vi "sumador encoder.vi"() -> ()   [LabVIEW 2025]
panel:
  out "Posición (flancos)":i32
  out "x+y":i32
  out "B":i32
  out "A":i32
  in  "stop":bool
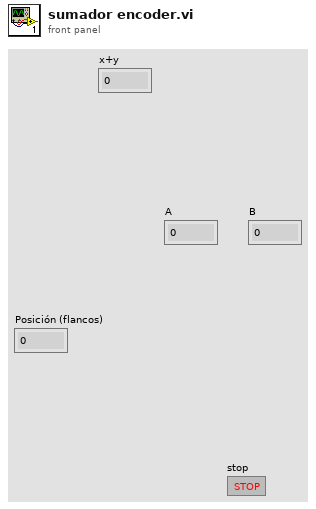
[diagram p1: front panel]
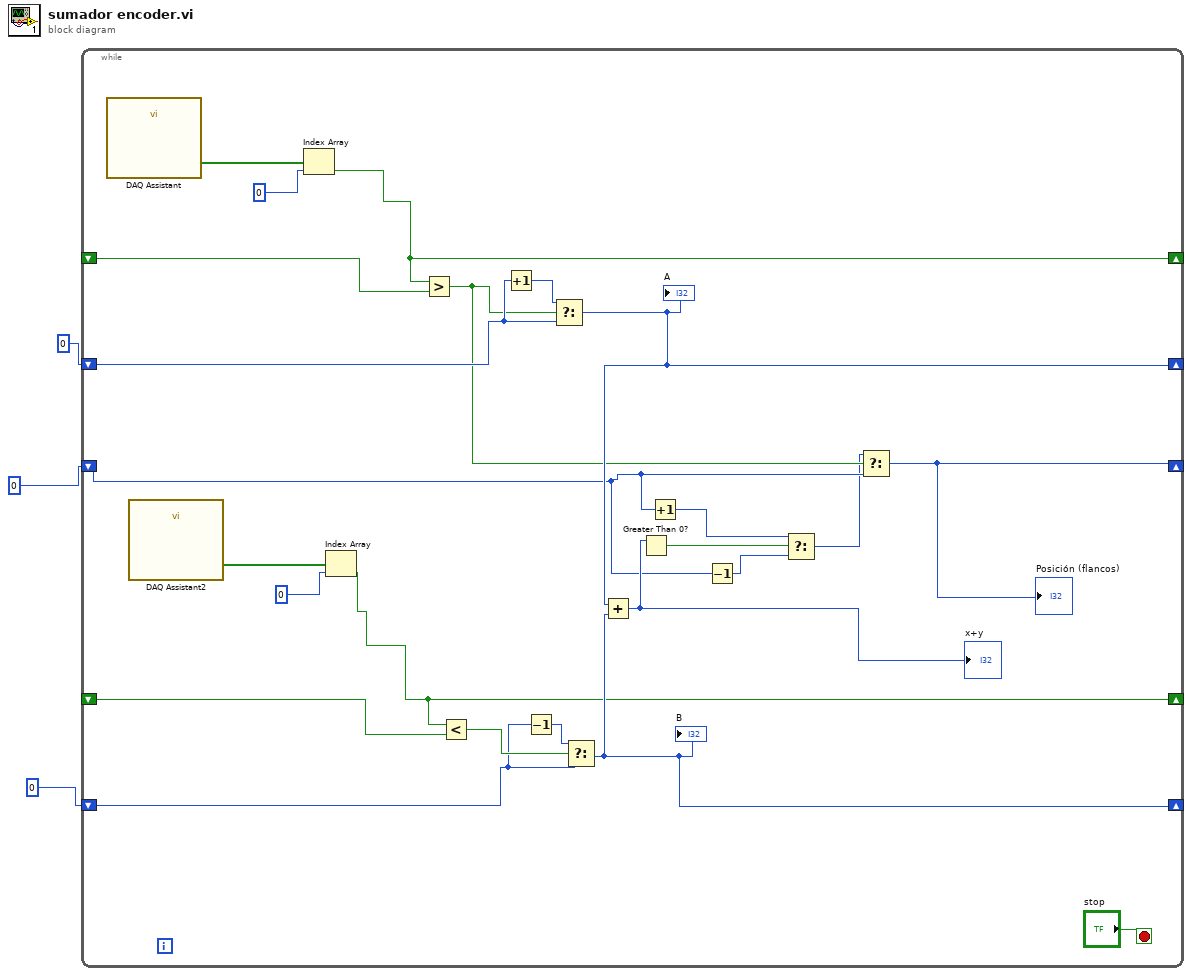
[diagram p0: block diagram]
diagram:
  n1 = while {
    shift-right: [w7] -> _
    shift-left: _ -> [w26]
    shift-right: [w18] -> _
    shift-left: 0 -> [w24]
    shift-right: [w4] -> _
    shift-left: _ -> [w23]
    shift-right: [w21] -> _
    shift-left: 0 -> [w19]
    shift-right: [w17] -> _
    shift-left: 0 -> [w12]
    stop <- "stop" stop-if-true
    n2 = call "DAQ Assistant"() -> ("data"=w9:bool[])  [unwired: 17 in, 2 out]
    n3 = call "DAQ Assistant2"() -> ("data"=w6:bool[])  [unwired: 17 in, 2 out]
    n4 = Index Array(array=w9, index=0) -> (element=w7:bool)
    n5 = Index Array(array=w6, index=0) -> (element=w4:bool)
    n6 = Greater?(x=w7, y=w26) -> (0:w16:bool)
    n7 = Less?(x=w4, y=w23) -> (x < y?=w22:bool)
    n8 = Increment(x=w24) -> (x+1=w25:i32)
    n9 = Decrement(x=w19) -> (x-1=w20:i32)
    n10 = Select(t=w25, s=w16, f=w24) -> (s? t:f=w18:i32)
    "A" <- w18
    n11 = Select(t=w20, s=w22, f=w19) -> (s? t:f=w21:i32)
    "B" <- w21
    n12 = Add(x=w18, y=w21) -> (x+y=w15:i32)
    "x+y" <- w15
    n13 = Greater Than 0?(x=w15) -> (x > 0?=w14:bool)
    n14 = Increment(x=w12) -> (x+1=w13:i32)
    n15 = Decrement(x=w12) -> (x-1=w11:i32)
    n16 = Select(t=w13, s=w14, f=w11) -> (s? t:f=w10:i32)
    n17 = Select(t=w10, s=w16, f=w12) -> (s? t:f=w17:i32)
    "Posición (flancos)" <- w17
  }
